vi "write_calibr_result_table.vi"(4 "new element/subarray":dbl[](array[numeric]), 5 "DC values":dbl, 6 "error in (no error)":errorcluster, 7 "index (col)":i32=-1, 8 "Enum":T4, 9 "UI in":T1) -> (0 "error out":errorcluster, 3 "UI_out":T1)   [LabVIEW 2017]
uses:
  ui.ctl
  classes/dc_power_supply/DC_power_supply.lvclass
  ui_buttons.ctl
  types/boc_type.ctl
  types/calibr_table_rows.ctl
  <vilib>/Utility/error.llb/DialogType.ctl
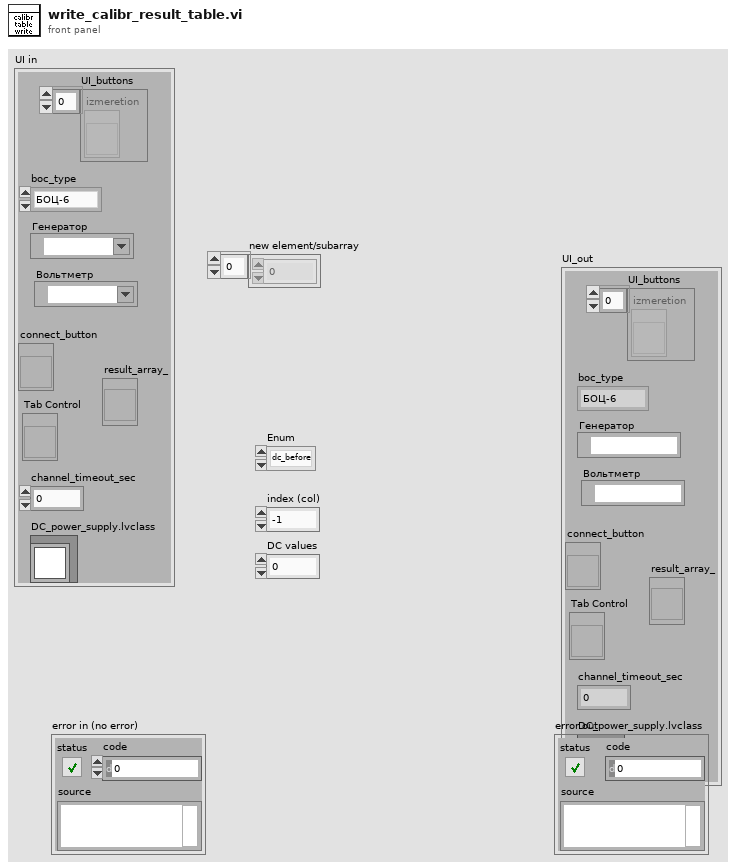
[diagram p1: front panel]
types:
  T1 = typedef "ui.ctl" = cluster{"UI_buttons":T2, "Tab Control":refnum<vi>, "connect_button":refnum<vi>, "generator":refnum<visa-resource-name>, "voltmetr":refnum<visa-resource-name>, "channel_timeout_sec":dbl, "boc_type":T3, "result_array_":refnum<vi>, "DC_power_supply.lvclass":refnum<class "DC_power_supply.lvclass">}
  T2 = typedef "ui_buttons.ctl" = refnum<vi>[]
  T3 = typedef "boc_type.ctl" = enum16{"БОЦ-6", "БОЦ-12"}
  T4 = typedef "calibr_table_rows.ctl" = enum16{"dc_before", "rms_before", "measured", "dc_result", "rms_result", "dc_after", "rms_after", "abs_before", "abs_after"}
  T5 = typedef "DialogType.ctl" = u16
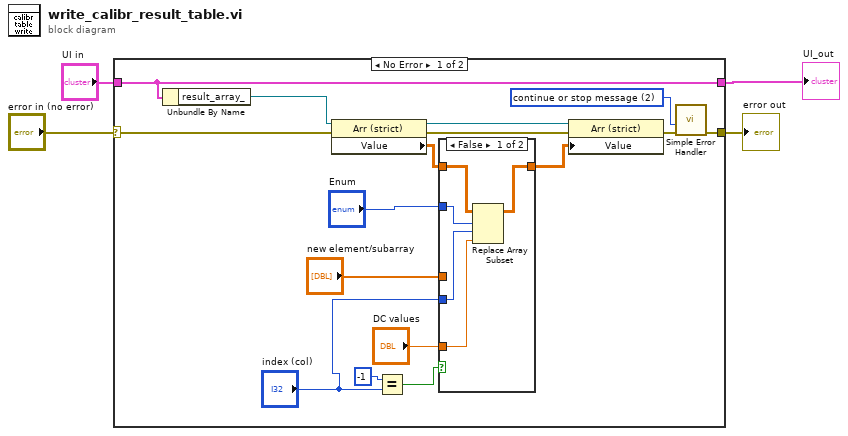
[diagram p0: block diagram]
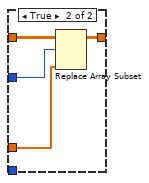
[diagram p2: hidden frame]
diagram:
  n1 = case shown="No Error" "error in (no error)" {
    selector: "error in (no error)" -> [w14 w30]
    tunnel: "UI in" -> [w13 w31]
    tunnel: [w11 w30] -> w4
    tunnel: [w13 w31] -> w2
    frame No Error {
      w10 = T5 2 items=["no dialog", "OK message", "continue or stop message", "OK message + warnings", "continue/stop + warnings"] ("type of dialog (OK msg:1)")
      n2 = Unbundle By Name(w13) -> ("result_array_"=w17:refnum<vi>)
      n3 = property class="Arr (strict)"(reference=w17, error in=w14) -> (reference out=w18:refnum<vi>, error out=w15:errorcluster, "Value"=w19:dbl[][])
      n4 = Equal?(x=-1, y="index (col)") -> (x = y?=w7:bool)
      n5 = case shown="False" w7 {
        tunnel: [w24 w29] -> w20
        tunnel: w19 -> [w23 w28]
        tunnel: "DC values" -> [w21 _]
        tunnel: "Enum" -> [w25 w27]
        tunnel: "new element/subarray" -> [_ w26]
        tunnel: "index (col)" -> [w22 _]
        frame False {
          n6 = Replace Array Subset(array=w23, new element=w21, index (row)=w25, index (col)=w22) -> (w24:dbl[][])
        }
        frame True {
          n7 = Replace Array Subset(array=w28, new element=w26, index (row)=w27) -> (w29:dbl[][])  [unwired: 1 in]
        }
      }
      n8 = property class="Arr (strict)"(reference=w18, error in=w15, "Value"=w20) -> (error out=w12:errorcluster)  [unwired: 1 out]
      n9 = call <vilib>:"Simple Error Handler.vi"("type of dialog (OK msg:1)"=w10, "error in (no error)"=w12) -> ("error out"=w11:errorcluster)  [unwired: 3 in, 4 out]
    }
    frame Error {
    }
  }
  "UI_out" <- w2
  "error out" <- w4
